vi "FixupVimsInProject.vi"(8 "error in (no error)":errorcluster) -> (0 "error out":errorcluster)   [LabVIEW 2020]
uses:
  vim-liner/vim-liner.lvlib
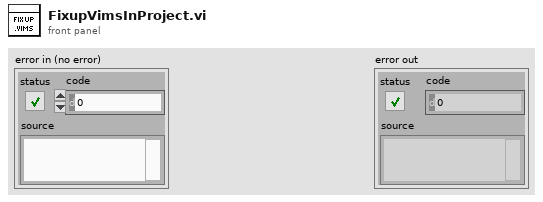
[diagram p1: front panel]
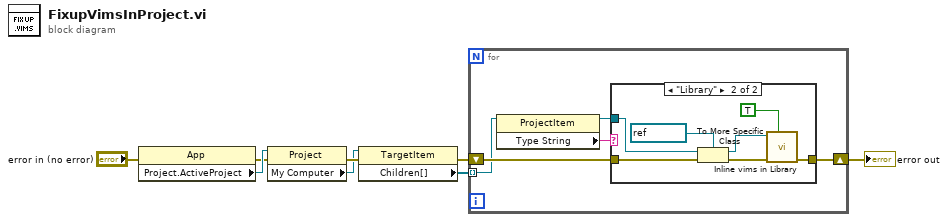
[diagram p0: block diagram]
diagram:
  n1 = property class="App"(error in="error in (no error)") -> (error out=w1:errorcluster, "Project.ActiveProject"=w3:refnum<vi>)  [unwired: 1 in, 1 out]
  n2 = property class="Project"(reference=w3, error in=w1) -> (error out=w6:errorcluster, "My Computer"=w5:refnum<vi>)  [unwired: 1 out]
  n3 = property class="TargetItem"(reference=w5, error in=w6) -> (error out=w4:errorcluster, "Children[]"=w7:refnum<vi>[])  [unwired: 1 out]
  n4 = for {
    shift-right: [w12] -> w8
    shift-left: w4 -> [w13]
    tunnel: w7 -> [w11] mode=indexing
    n5 = property class="ProjectItem"(reference=w11) -> (reference out=w9:refnum<vi>, "Type String"=w10:string)  [unwired: 1 in, 1 out]
    n6 = case shown="\"Library\"" w10 {
      tunnel: w13 -> [w14 w17]
      tunnel: [w14 w21] -> w12
      tunnel: w9 -> [_ w19]
      frame Default {
      }
      frame "Library" {
        n7 = To More Specific Class(target class=refnum<vi> refnum ("Library"), reference=w19, error in=w17) -> (specific class reference=w15:refnum<vi>, error out=w16:errorcluster)
        n8 = call "Inline vims in Library.vi"("Just Fixup"=TRUE, "error in"=w16, "Library"=w15) -> ("error out"=w21:errorcluster)  [unwired: 8 in]
      }
    }
  }
  "error out" <- w8
